vi "TR_SW_Gen_Get_Initial_picture_Scaling_and_Cage_size_DAQmx.vi"(7 "Input cluster of parameters":T3={"Cage diameter, mm"=180, "Starting angle MIDFIELD"=0, "Starting angle BORDER"=0, "Radius, mm CENTER"=30, "Radius, mm MIDFIELD"=60, "N segments MIDFIELD"=4, "N segments BORDER"=8, "R-gap, mm"=0.0, "Bridge swap"=FALSE, "Bridge H. offset"=0.0, "Bridge V. offset"=0.0, "Twisted neck"=FALSE, "Alt. magn. orientation"=FALSE, "Sensor board size"=enum."Small"} {"Cage diameter, mm" scale=0.0..340.0}, 8 "Error In":errorcluster, 9 "Scale factor for outer display radius display":dbl=0.95 format="%#_13g", 10 "Background color":u32(colorbox)=13816530, 11 "Draw Area Size":T4={"Width"=480, "Height"=480}) -> (0 "Error Out":errorcluster, 1 "Width of the borders combined out":cluster{"Width":i32, "Height":i32}, 2 "Image geometrical and scaling parameters":T2, 3 "Background Image":T1(plugin-control))   [LabVIEW 2018, in "Tracks Repair.lvlib"]
uses:
  Tracks Repair.lvlib
  SubVi's/Controls/CTL_Draw_Area_Size.ctl
  SubVi's/Controls/CTL_Segmented_plot_parameters.ctl
  SubVi's/Controls/CTL_Image_Geometrical_and_scaling_parameters.ctl
  Common_Resources.lvlib
panel:
  in  "Width of the borders combined":cluster{"Width":i32, "Height":i32}
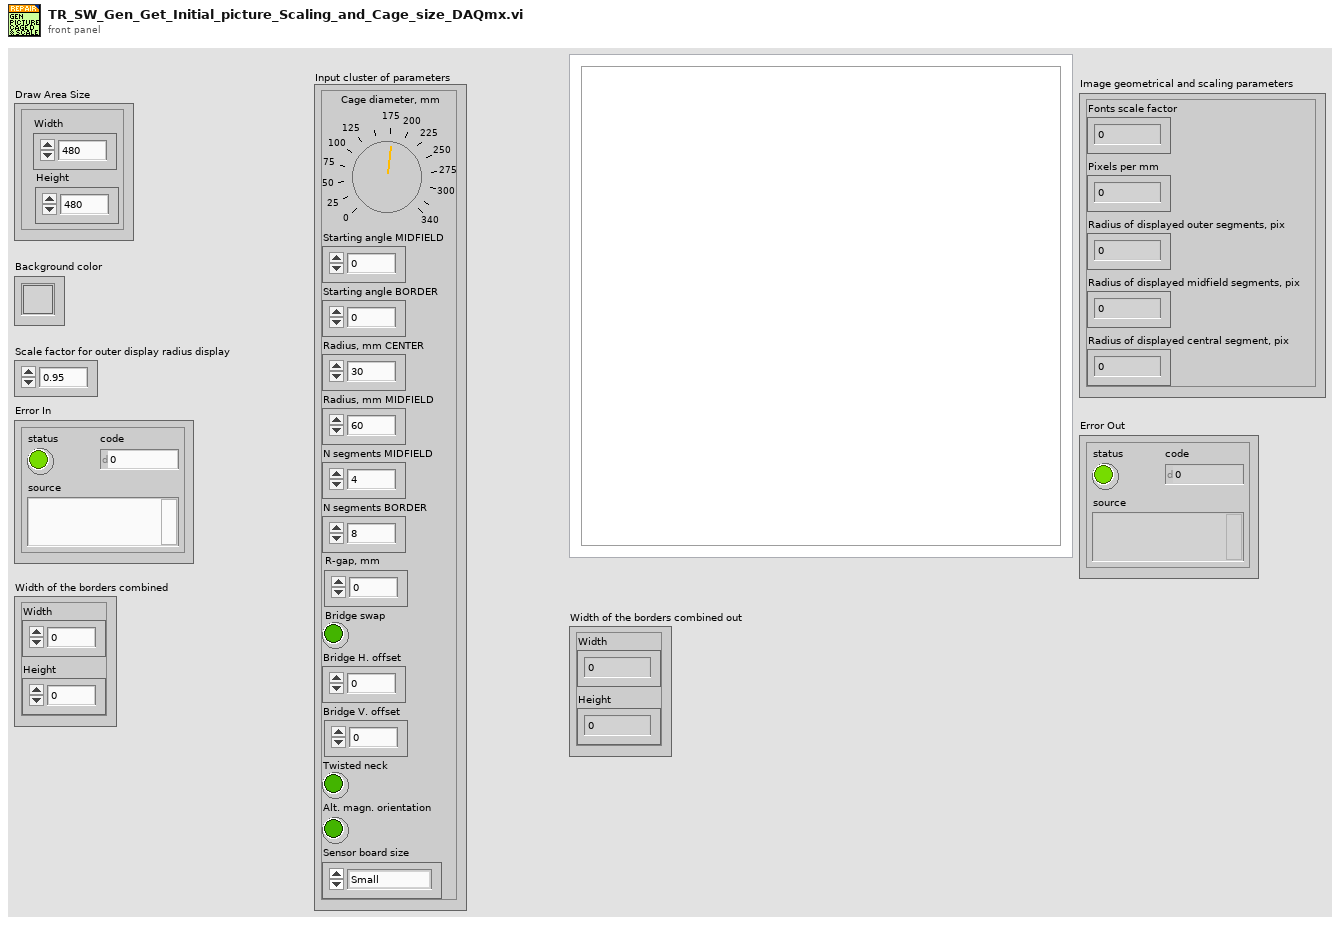
[diagram p1: front panel]
types:
  T1 = typedef "IMAQ Image.ctl" = refnum<image>
  T2 = typedef "Common_Resources.lvlib/CTL_Image_Geometrical_and_scaling_parameters.ctl" = cluster{"Fonts scale factor":dbl, "Pixels per mm":dbl, "Radius of displayed outer segments, pix":dbl, "Radius of displayed midfield segments, pix":dbl, "Radius of displayed central segment, pix":dbl}
  T3 = typedef "Common_Resources.lvlib/CTL_Segmented_plot_parameters.ctl" = cluster{"Cage diameter, mm":u16, "Starting angle MIDFIELD":i16, "Starting angle BORDER":i16, "Radius, mm CENTER":u16, "Radius, mm MIDFIELD":u16, "N segments MIDFIELD":u8, "N segments BORDER":u8, "R-gap, mm":sgl, "Bridge swap":bool, "Bridge H. offset":sgl, "Bridge V. offset":sgl, "Twisted neck":bool, "Alt. magn. orientation":bool, "Sensor board size":enum16{"Small", "Large"}}
  T4 = typedef "Common_Resources.lvlib/CTL_Draw_Area_Size.ctl" = cluster{"Width":i32, "Height":i32}
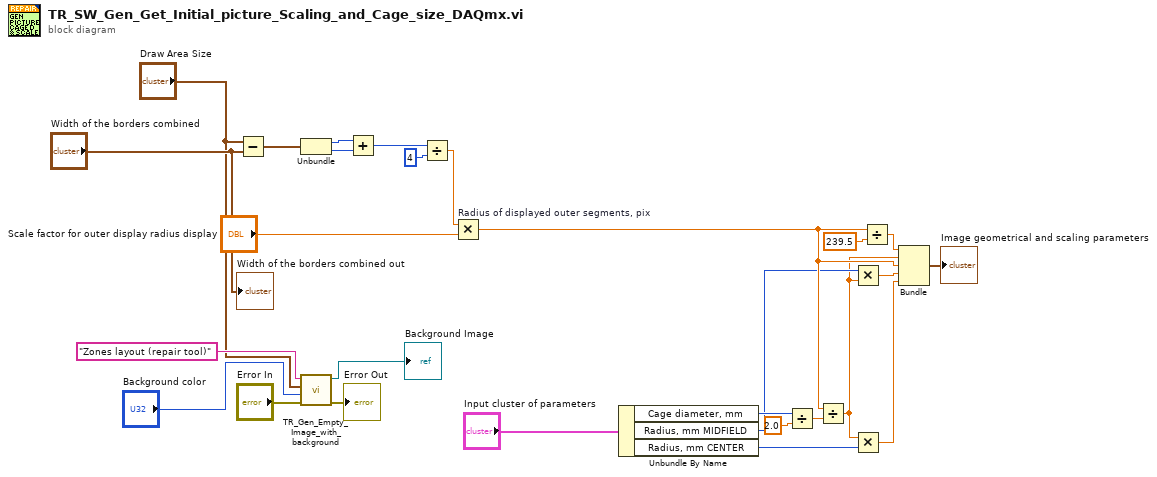
[diagram p0: block diagram]
diagram:
  n1 = Subtract(x="Draw Area Size", y="Width of the borders combined") -> (x-y=w19:T4)
  n2 = Unbundle(w19) -> ("Width"=w26:i32, "Height"=w27:i32)
  n3 = call "TR_Gen_Empty_Image_with_background.vi"("error in (no error)"="Error In", "Background color"="Background color", "Draw Area Size (480 x 480)"="Draw Area Size", "Image Name"="Zones layout (repair tool)") -> ("error out"=→"Error Out":errorcluster, "Image refnum out"=→"Background Image":T1)  [unwired: 6 in]
  n4 = Add(x=w26, y=w27) -> (x+y=w25:i32)
  n5 = Divide(x=w25, y=u32 4) -> (x/y=w22:dbl)
  n6 = Multiply "Radius of displayed outer segments, pix"(x=w22, y="Scale factor for outer display radius display") -> (x*y=w13:dbl)
  n7 = Unbundle By Name("Input cluster of parameters") -> ("Cage diameter, mm"=w15:u16, "Radius, mm MIDFIELD"=w12:u16, "Radius, mm CENTER"=w10:u16)
  n8 = Divide(x=w15, y=2.0) -> (x/y=w17:dbl)
  n9 = Divide(x=w13, y=w17) -> (x/y=w11:dbl)
  n10 = Multiply(x=w12, y=w11) -> (x*y=w9:dbl)
  n11 = Multiply(x=w11, y=w10) -> (x*y=w8:dbl)
  n12 = Divide(x=w13, y=239.5) -> (x/y=w14:dbl)
  n13 = Bundle(w14, w11, w13, w9, w8) -> (→"Image geometrical and scaling parameters":cluster{dbl, dbl, dbl, dbl, dbl})  [unwired: 1 in]
  "Width of the borders combined out" <- "Width of the borders combined"
